vi "Convert string to DBL or DBL to string (simple).vi"(6 "Format":string="%<%Ss%3ums>t", 9 "Number in (DBL)":dbl, 10 "String in":string, 11 "Mode":enum16{"String to Number", "Number to String"}(ring)) -> (1 "String out":string, 2 "Number out(DBL)":dbl)   [LabVIEW 2020]
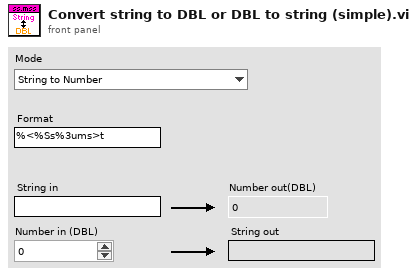
[diagram p1: front panel]
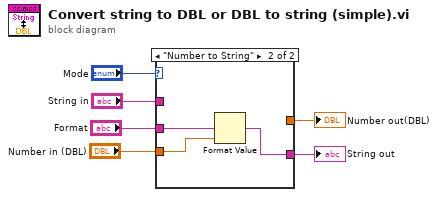
[diagram p0: block diagram]
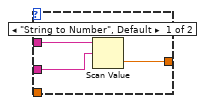
[diagram p2: hidden frame]
diagram:
  n1 = case shown="\"Number to String\"" "Mode" {
    tunnel: "Format" -> [w9 w12]
    tunnel: [w8 _] -> w5
    tunnel: "String in" -> [w7 _]
    tunnel: "Number in (DBL)" -> [_ w11]
    tunnel: [_ w10] -> w1
    frame "String to Number", Default {
      n2 = Scan Value(string=w7, format string=w9) -> (value=w8:dbl)  [unwired: 1 in, 1 out]
    }
    frame "Number to String" {
      n3 = Format Value(format string=w12, value (0)=w11) -> (output string=w10:string)  [unwired: 1 in]
    }
  }
  "Number out(DBL)" <- w5
  "String out" <- w1
